vi "Robot Global Data.vi"() -> ()   [LabVIEW 2011]
doc: "This global VI can contain as many global variables as you need. Place a control on the panel, give it a good name. To read or write to it from a VI, drag the icon to the diagram of that VI. You can also drag from the project. Click on the node to change which global you access. You shouldn't have multiple locations writing to a global or it will cause a race-condition."
panel:
  out "Bad Shot":bool
  out "Max":bool=TRUE
  out "Poop":bool=TRUE
  out "Encoder Right Rate":dbl
  out "Encoder Left Rate":dbl
  out "Turret Button 5":bool
  out "Turret Button 4":bool
  out "Shoot All":bool
  in  "SpinerOptions":enum16{"Full", "16", "14", "12", "Poop"}(ring)=enum."14"
  in  "BallActionNew":T1(ring)
  out "Encoder3 Rate":dbl
  out "Motor Reverse":bool
  out "Setpoint Start Enc":dbl
  out "Top-X":dbl
  in  "EncoderRight":dbl
  in  "EncoderLeft":dbl
  out "Tipper Buttons":i32
  out "Shoot":bool
  out "Turret Joystick X-Axis":dbl
  out "Manual/Auto":bool
  out "Load":bool
  out "Balance Motor Speed":dbl
  out "14 Foot":bool=TRUE
  out "12 Foot":bool=TRUE
  out "16 Foot":bool=TRUE
  out "Selected Target Distance":dbl
  out "Tacometer":dbl
  out "Encoder4 Rate":dbl
  out "Top45":dbl[](array[numeric])=[-0.0, nan, nan, nan, nan, nan, nan, nan, nan, nan, nan, nan, nan, nan, nan, nan, nan, nan, nan, nan, nan, nan, nan, nan, nan, nan, nan, nan, nan, nan, nan, nan, 1883.5199604911154, 617.7924513800123, 461.9166339564075, 391.7400478505252, 350.53788058796005, 323.12530022428314, 303.5011842794952, 288.76192837202757, 277.3123944399277, 268.19573643797355, 260.7995983067292, 254.71208752156898, 249.6449840249085, 245.3900171210353, 241.79261797258053, 238.7354610224012, 236.12775931033894, 233.89808200074404, 231.98940410935217, 230.35561397453648, 228.9589980062319, 227.76839593038605, 226.75782559893628, 225.90544274893503, 225.19274367211108, 224.6039467040343, 224.12550715645853, 223.74573307686308, 223.45447806480396, 223.24289359992994, 223.1032277789923, 223.0286605703624, 223.01316804346058, 223.05140976769397, 223.1386348735432, 223.27060324768053, 223.44351907938636, 223.65397454769052, 223.8989018813374, 224.17553236871257, 224.48136116569924, 224.81411696342477, 225.17173574800017, 225.55233802043867, 225.95420895439426, 226.37578105787162, 226.81561897699387, 227.2724061386666, 227.7449329771796, 228.23208652951237, 228.73284121698637, 229.24625065822198, 229.77144038114602, 230.3076013208721, 230.85398400630498, 231.40989335183292, 231.97468398190236, 232.54775602596757, 233.12855132956125, 233.7165500342784, 234.31126748549434, 234.9122514318157, 235.51907948471572, 236.13135681064796, 236.74871403125562, 237.37080531017475, 237.99730660743143, 238.62791408461288, 239.26234264589465, 239.90032460166785, 240.54160844296874, 241.18595771619067, 241.83314998868536, 242.48297589684975, 243.13523826917182, 243.78975131748126, 244.44633989033713, 245.10483878309222, 245.76509209971513, 246.42695266193095, 247.09028146167122, 247.75494715320588, 248.42082558167198, 249.0877993450208, 249.75575738667928, 250.4245946164668, 251.09421155753267, 251.76451401727547, 252.435412780388, 253.10682332233108, 253.77866554168781, 254.45086350998022, 255.1233452376515, 255.79604245502446, 256.4688904071455, 257.1418276615132, 257.814795927771, 258.48773988851775, 259.1606070404576, 259.8333475451714, 260.5059140888477, 261.1782617503634, 261.85034787715006, 262.52213196832474, 263.1935755646037, 263.864642144553, 264.53529702676326, 265.205507277565, 265.87524162393015, 266.54447037123055, 267.2131653255461, 267.8812997202396, 268.54884814653354, 269.21578648784134, 269.882091857626, 270.5477425405716, 271.21271793686867, 271.87699850942766, 272.54056573384855, 273.2034020509831, 273.86549082193994, 274.52681628539085, 275.187363517046, 275.8471183911745, 276.5060675440549, 277.16419833924675, 277.82149883458203, 278.4779577507806, 279.13356444160104, 279.7883088654424, 280.44218155831805, 281.0951736081287, 281.74727663016273, 282.39848274376186, 283.0487845500869, 283.69817511092856, 284.3466479285075, 284.99419692621245, 285.6408164302286, 286.28650115200946, 286.9312461715505, 287.5750469214238, 288.2178991715341, 288.8597990145623, 289.5007428520605, 290.1407273811669, 290.77974958191066, 291.4178067050771, 292.0548962606063, 292.69101600649975, 293.3261639382098, 293.9603382784894, 294.5935374676806, 295.2257601544201, 295.85700518674247, 296.4872716035642, 297.11655862652736, 297.7448656521901, 298.3721922445447, 298.9985381278508, 299.6239031797675, 300.24828742477206, 300.87169102785117, 301.4941142884539, 302.11555763469306, 302.73602161778547, 303.3555069067191, 303.97401428313844, 304.59154463643733, 305.2080989590511, 305.82367834193883, 306.4382839702477, 307.0519171191515, 307.66457914985597, 308.2762715057637, 308.88699570879174, 309.49675335583584, 310.1055461153745, 310.71337572420765, 311.32024398432384, 311.92615275989044, 312.5311039743629, 313.1350996077065, 313.7381416937267, 314.3402323175046, 314.94137361293144, 315.5415677603392, 316.1408169842232, 316.7391235510533, 317.33648976716944, 317.93291797675823, 318.52841055990865, 319.12296993074125, 319.7165985356107, 320.3092988513765, 320.9010733837409, 321.49192466564983, 322.0818552557557, 322.67086773693893, 323.25896471488596, 323.8461488167222, 324.4324226896964, 325.0177889999165, 325.6022504311325, 326.18580968356736, 326.768469472791, 327.3502325286391, 327.93110159417137, 328.5110794246717, 329.09016878668484, 329.6683724570912, 330.24569322221646, 330.8221338769757, 331.3976972240504, 331.9723860730965, 332.5462032399844, 333.1191515460664, 333.69123381747403, 334.2624528844418, 334.83281158065734, 335.40231274263664, 335.97095920912403, 336.53875382051524, 337.10569941830323, 337.6717988445456, 338.23705494135316, 338.80147055039856, 339.3650485124446, 339.9277916668912, 340.48970285134, 341.05078490117734, 341.6110406491734, 342.17047292509756, 342.72908455534963, 343.2868783626061, 343.84385716548064, 344.40002377819894, 344.9553810102868, 345.5099316662717, 346.06367854539616, 346.61662444134396, 347.16877214197757, 347.72012442908715, 348.2706840781503, 348.82045385810176, 349.3694365311147, 349.9176348523898, 350.46505156995545, 351.01168942447595, 351.55755114906884, 352.1026394691309, 352.6469571021717, 353.1905067576556, 353.7332911368512, 354.2753129326878, 354.816574829619, 355.35707950349365, 355.8968296214326, 356.4358278417122, 356.974076813654, 357.51157917751993, 358.0483375644139, 358.5843545961876, 359.11963288535327, 359.6541750350003, 360.1879836387171, 360.72106128051803, 361.25341053477433, 361.78503396615037, 362.315934129543, 362.846113570026, 363.37557482279783, 363.90432041313386, 364.43235285634137, 364.95967465771923, 365.4862883125199, 366.0121963059155, 366.5374011129669, 367.06190519859535, 367.58571101755814, 368.1088210144258, 368.63123762356327, 369.1529632691127, 369.6740003649798, 370.1943513148215, 370.71401851203706, 371.23300433976067, 371.7513111708568, 372.268941367917, 372.7858972832599, 373.3021812589314, 373.8177956267087, 374.33274270810455, 374.8470248143741, 375.3606442465234, 375.873603295319, 376.38590424129956, 376.8975493547888, 377.40854089590994, 377.91888111460133, 378.42857225063375, 378.9376165336285, 379.4460161830771, 379.95377340836205, 380.46089040877865, 380.9673693735578, 381.47321248189024, 381.97842190295114, 382.4829997959263, 382.98694831003877, 383.4902695845765, 383.9929657489208, 384.4950389225759, 384.99649121519855, 385.497324726629, 385.9975415469227, 386.4971437563817, 386.99613342558825, 387.4945126154374, 387.9922833771713, 388.48944775241364, 388.98600777320445, 389.48196546203553, 389.9773228318867, 390.4720818862615, 390.96624461922477, 391.4598130154392, 391.95278905020285]
  out "Encoder 7 aDistance":dbl
  out "Setpoint End":dbl
  in  "LED toggle rate (ms)":u32=100
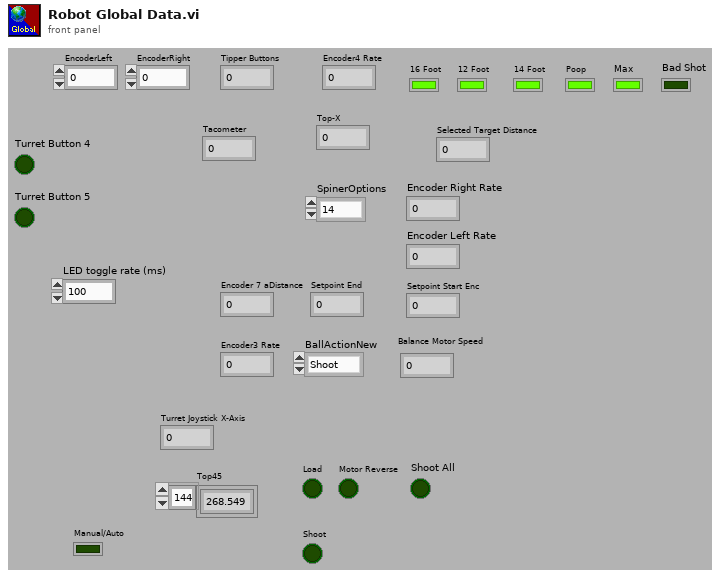
[diagram p1: front panel]
types:
  T1 = enum16{"Shoot", "Load", "Arm", "Nothing", "Reverse", "ShootAll"}
diagram:
